vi "DataBlock_Panel_Rev11.vi"(2 "error in":errorcluster, 3 "Run Data SubPanel Input":T1) -> (0 "error out":errorcluster, 1 "Run Data SubPanel Output":T1)   [LabVIEW 2019]
uses:
  Controls/DataBlockControl.ctl
panel:
  out "Changes Applied?":bool
  in  "Run Data Input":T1={"Run Folder Parent Directory"=path "C:/Data/dump", "DUT"="None", "Ion (ex Kr)"="None", "Board Number"="NA", "Effective LET"="0", "Test Type"=enum."Single Event Latchup"}
  out "Confirmed FilePath":path
  in  "Return to control panel":bool
  in  "Apply Data":bool
  out "DUT Indicator":string
  out "Ion Indicator":string
  out "Board Number Indicator":string
  out "Effective LET Indicator":string
  out "Test Type Indicator":string="SEL"
  # "Instructions:\nIn the \"Run Data Input\" block, input the following parameters:\n\nRun Folder Parent Directory: The main folder where runs will be stored. You must already have this folder created (preferably empty)\n\nDUT: Device under test\n\nIon (ex Kr): Ion that we are using\n\nBoard Number: User defined number of the board that is tested (typically written in sharpie on the eval board\n\nEffective LET: linear energy transfer that we are testing. Related to the ion. \n\nOnce data is inputted, press \"Apply Data\" button\n\nReview the \"OUTPUT ECHO\" to confirm that what you inputted is correct\n\nPress \"EXIT\" to complete this configuration"
  # "Nothing behind here, surely"
  # "IMPORTANT NOTE: \nThis code automatically increments the runs based off the amount of folders it detects within the \"Run Folder Parent Directory\" (i.e. if there are two folders already in there, it would begin run three). You must account for this if you are not starting from run 1"
  # "OUTPUT ECHO"
  # "CHANGES APPLIED? MUST BE BRIGHT GREEN BEFORE EXITING"
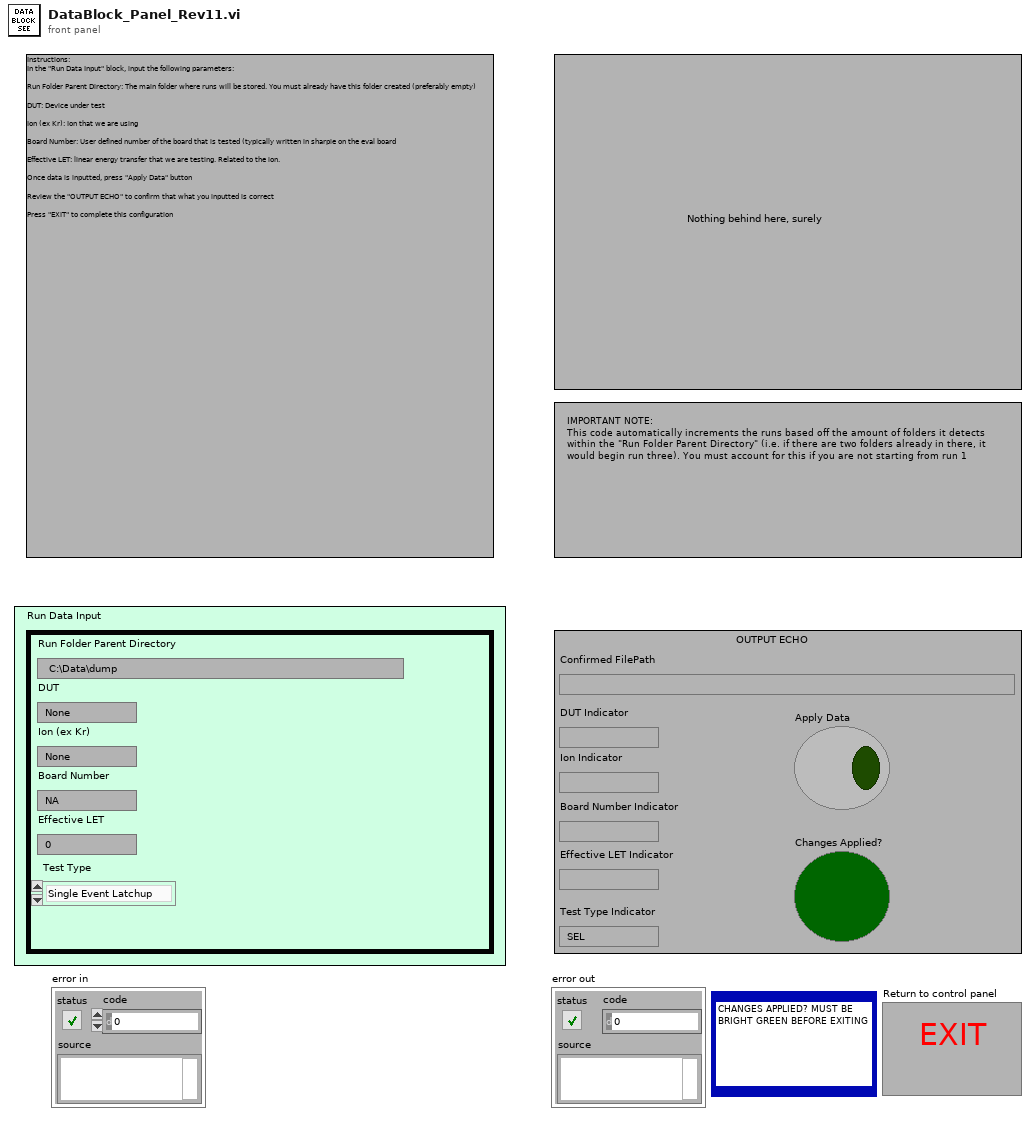
[diagram p1: front panel]
types:
  T1 = typedef "DataBlockControl.ctl" = cluster{"Run Folder Parent Directory":path, "DUT":string, "Ion (ex Kr)":string, "Board Number":string, "Effective LET":string, "Test Type":enum16{"Single Event Latchup", "Single Event Transient", "Single Event Upset"}}
  T2 = cluster{"Run Folder Parent Directory":bool, "DUT":bool, "Ion (ex Kr)":bool, "Board Number":bool, "Effective LET":bool, "Test Type":bool}
  T3 = enum16{"Single Event Latchup", "Single Event Transient", "Single Event Upset"}
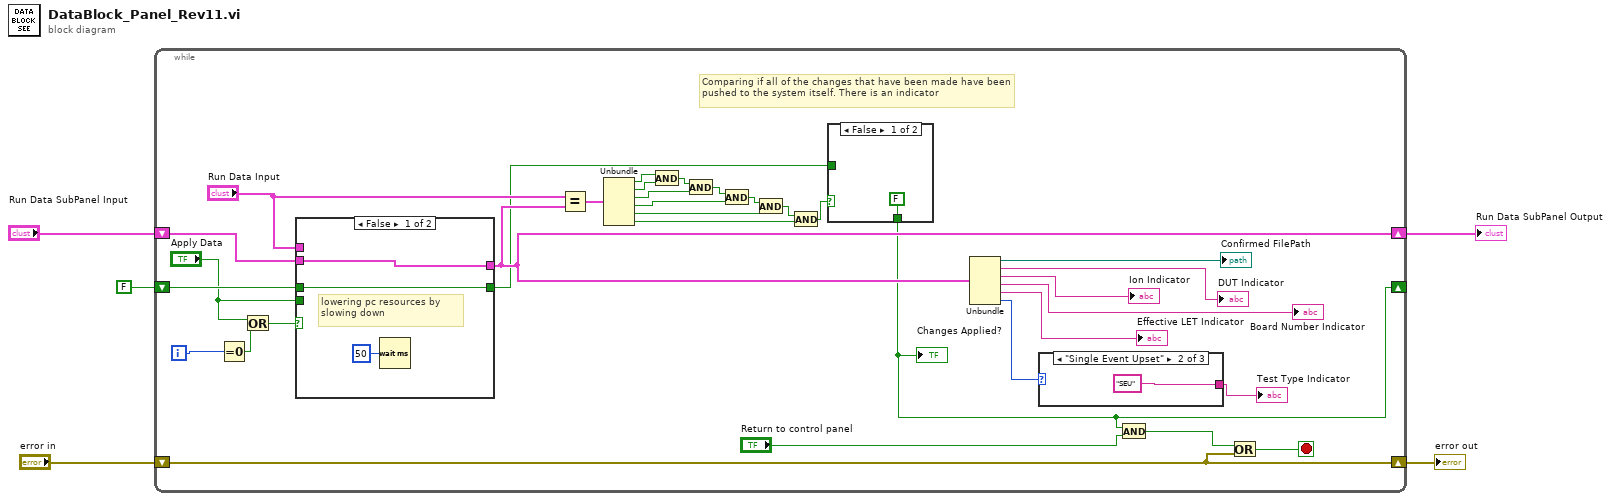
[diagram p0: block diagram]
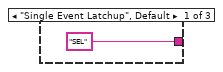
[diagram p3: hidden frame]
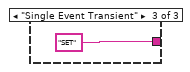
[diagram p4: hidden frame]
diagram:
  n1 = while {
    shift-right: [w23] -> w4
    shift-left: "Run Data SubPanel Input" -> [w35]
    shift-right: [w26] -> w2
    shift-left: "error in" -> [w26]
    shift-right: [w8] -> _
    shift-left: FALSE ("Apply Data") -> [w25]
    i -> [w37]
    stop <- w27 stop-if-true
    # "Comparing if all of the changes that have been made have been pushed to the system itself. There is an indicator"
    n2 = Equal To 0?(x=w37) -> (x = 0?=w36:bool)
    n3 = Or(x="Apply Data", y=w36) -> (x .or. y?=w38:bool)
    n4 = case shown="False" w38 {
      tunnel: [w46 w47] -> w23
      tunnel: w35 -> [w46 _]
      tunnel: w25 -> [w44 _]
      tunnel: [w44 w48] -> w21
      tunnel: "Apply Data" -> [_ w48]
      tunnel: "Run Data Input" -> [_ w47]
      frame False {
        # "lowering pc resources by slowing down"
        n5 = Wait (ms)(milliseconds to wait=u32 50) -> ()  [unwired: 1 out]
      }
      frame True {
      }
    }
    n6 = Equal?(x="Run Data Input", y=w23) -> (x = y?=w20:T2)
    n7 = Unbundle(w20) -> ("Run Folder Parent Directory"=w16:bool, "DUT"=w15:bool, "Ion (ex Kr)"=w14:bool, "Board Number"=w13:bool, "Effective LET"=w12:bool, "Test Type"=w10:bool)
    n8 = And(x=w16, y=w15) -> (x .and. y?=w19:bool)
    n9 = And(x=w19, y=w14) -> (x .and. y?=w17:bool)
    n10 = And(x=w17, y=w13) -> (x .and. y?=w18:bool)
    n11 = And(x=w18, y=w12) -> (x .and. y?=w11:bool)
    n12 = And(x=w11, y=w10) -> (x .and. y?=w9:bool)
    n13 = case shown="False" w9 {
      tunnel: w21 -> [_ w40]
      tunnel: [FALSE ("Apply Data") w40] -> w8
      frame False {
      }
      frame True {
      }
    }
    "Changes Applied?" <- w8
    n14 = Unbundle(w23) -> ("Run Folder Parent Directory"=→"Confirmed FilePath":path, "DUT"=→"DUT Indicator":string, "Ion (ex Kr)"=→"Ion Indicator":string, "Board Number"=→"Board Number Indicator":string, "Effective LET"=→"Effective LET Indicator":string, "Test Type"=w29:T3)
    n15 = case shown="\"Single Event Upset\"" w29 {
      tunnel: ["SEL" "SEU" "SET"] -> w28
      frame "Single Event Latchup", Default {
      }
      frame "Single Event Upset" {
      }
      frame "Single Event Transient" {
      }
    }
    "Test Type Indicator" <- w28
    n16 = And(x=w8, y="Return to control panel") -> (x .and. y?=w6:bool)
    n17 = Or(x=w6, y=w26) -> (x .or. y?=w27:bool)
  }
  "Run Data SubPanel Output" <- w4
  "error out" <- w2
